vi "Escape Reserve Word.vi"(8 "error in (no error)":errorcluster, 10 "Input Name":string, 11 "MS Access Database Engine in":refnum<class "MS Access Database Engine.lvclass">) -> (0 "error out":errorcluster, 2 "Escaped Name":string, 3 "MS Access Database Engine out":refnum<class "MS Access Database Engine.lvclass">)   [LabVIEW 2020, in "ADODB.lvlib" / "MS Access Database Engine.lvclass"]
uses:
  MS Access Database Engine.lvclass
  MS Access Reserved Words.ctl
panel:
  # "The method takes an input name and checks it against a reserve word list. \n-If the name is reserved, this method attempts to add escape characters to allow for a valid SQL query\n-If escaping the word is not possible, this method returns an error\n-If the the name is not reserved, the method returns a copy of the name"
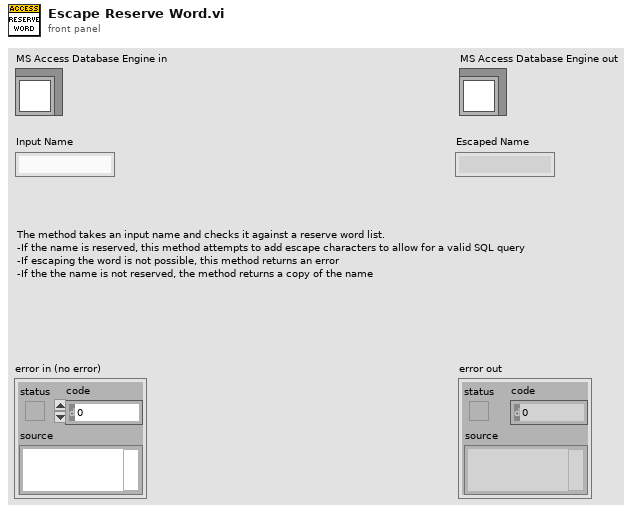
[diagram p1: front panel]
types:
  T1 = typedef "ADODB.lvlib/MS Access Database Engine.lvclass/MS Access Reserved Words.ctl" = set{string}
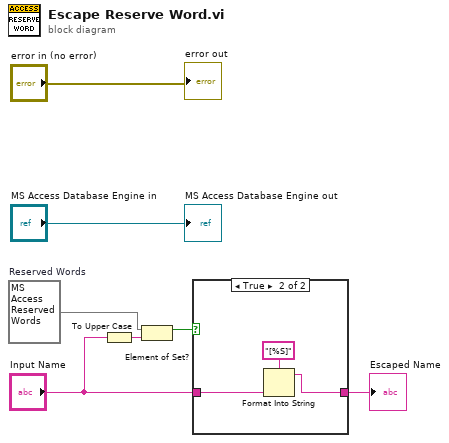
[diagram p0: block diagram]
diagram:
  w5 = T1 {"", "ABSOLUTE", "ADD", "ADMINDB", "ALL", "ALPHANUMERIC", "ALTER", "ALTER TABLE", "AND", "ANY", "ARE", "AS", "ASC", "ASSERTION", "AUTHORIZATION", "AUTOINCREMENT", "AVG", "BEGIN", "BETWEEN", "BINARY", "BIT", "BIT_LENGTH", "BOOLEAN", "BOTH", "BY", "BYTE", "CASCADE", "CATALOG", "CHAR", "CHARACTER", "CHARACTER_LENGTH", "CHAR_LENGTH", "CHECK", "CLOSE", "CLUSTERED", "COALESCE", "COLLATE", "COLLATION", "COLUMN", "COMMIT", "COMP", "COMPRESSION", "CONNECT", "CONNECTION", "CONSTRAINT", "CONSTRAINTS", "CONTAINER", "CONTAINS", "CONVERT", "COUNT", "COUNTER", "CREATE", "CURRENCY", "CURRENT_DATE", "CURRENT_TIME", "CURRENT_TIMESTAMP", "CURRENT_USER", "CURSOR", "DATABASE", "DATE", "DATETIME", "DAY", "DEC", "DECIMAL", "DECLARE", "DELETE", "DESC", "DISALLOW", "DISCONNECT", "DISTINCT", "DISTINCTROW", "DOMAIN", "DOUBLE", "DROP", "EQV", "EXCLUSIVECONNECT", "EXEC", "EXECUTE", "EXISTS", "EXTRACT", "FALSE", "FETCH", "FIRST", "FLOAT", "FLOAT4", "FLOAT8", "FOREIGN", "FROM", "GENERAL", "GRANT", "GROUP", "GUID", "HAVING", "HOUR", "IDENTITY", "IEEEDOUBLE", "IEEESINGLE", "IGNORE", "IMAGE", "IMP", "IN", "INDEX", "INDEXCREATEDB", "INNER", "INPUT", "INSENSITIVE", "INSERT", "INSERT INTO", "INT", "INTEGER", "INTEGER1", "INTEGER2", "INTEGER4", "INTERVAL", "INTO", "IS", "ISOLATION", "JOIN", "KEY", "LANGUAGE", "LAST", "LEFT", "LEVEL", "LIKE", "LOGICAL", "LOGICAL1", "LONG", "LONGBINARY", "LONGCHAR", "LONGTEXT", "LOWER", "MATCH", "MAX", "MEMO", "MIN", "MINUTE", "MOD", "MONEY", "MONTH", "NATIONAL", "NCHAR", "NONCLUSTERED", "NOT", "NTEXT", "NULL", "NUMBER", "NUMERIC", "NVARCHAR", "OCTET_LENGTH", "OLEOBJECT", "ON", "OPEN", "OPTION", "OR", "ORDER", "OUTER", "OUTPUT", "OWNERACCESS", "PAD", "PARAMETERS", "PARTIAL", "PASSWORD", "PERCENT", "PIVOT", "POSITION", "PRECISION", "PREPARE", "PRIMARY", "PRIVILEGES", "PROC", "PROCEDURE", "PUBLIC", "REAL", "REFERENCES", "RESTRICT", "REVOKE", "RIGHT", "ROLLBACK", "SCHEMA", "SECOND", "SELECT", "SELECTSCHEMA", "SELECTSECURITY", "SET", "SHORT", "SINGLE", "SIZE", "SMALLDATETIME", "SMALLINT", "SMALLMONEY", "SOME", "SPACE", "SQL", "SQLCODE", "SQLERROR", "SQLSTATE", "STDEV", "STDEVP", "STRING", "SUBSTRING", "SUM", "SYSNAME", "SYSTEM_USER", "TABLE", "TABLEID", "TEMPORARY", "TEXT", "TIME", "TIMESTAMP", "TIMEZONE_HOUR", "TIMEZONE_MINUTE", "TINYINT", "TO", "TOP", "TRAILING", "TRANSACTION", "TRANSFORM", "TRANSLATE", "TRANSLATION", "TRIM", "TRUE", "UNION", "UNIQUE", "UNIQUEIDENTIFIER", "UNKNOWN", "UPDATE", "UPDATEIDENTITY", "UPDATEOWNER", "UPDATESECURITY", "UPPER", "USAGE", "USER", "USING", "VALUE", "VALUES", "VAR", "VARBINARY", "VARCHAR", "VARP", "VARYING", "VIEW", "WHEN", "WHENEVER", "WHERE", "WITH", "WORK", "XOR", "YEAR", "YESNO", "ZONE"}  # Reserved Words
  n1 = To Upper Case(1:"Input Name") -> (0:w4:string)
  n2 = Element of Set?(10:w4, 11:w5) -> (3:w3:bool)
  n3 = case shown="True" w3 {
    tunnel: "Input Name" -> [w8 w10]
    tunnel: [w8 w9] -> w1
    frame False {
    }
    frame True {
      n4 = Format Into String(format string="[%S]", w10) -> (resulting string=w9:string)  [unwired: 2 in, 1 out]
    }
  }
  "Escaped Name" <- w1
  "error out" <- "error in (no error)"
  "MS Access Database Engine out" <- "MS Access Database Engine in"
